vi "S2C_5190CR_Proc_SetOutput.vi"(7 "Local?":bool, 8 "Error In":errorcluster, 10 "Command":string, 11 "JSON String":string) -> (0 "Error Out":errorcluster, 3 "Response":variant)   [LabVIEW 2015]
doc: "Configures the state of an outlet."
uses:
  S2C_5190CR_Proc_Globals.vi
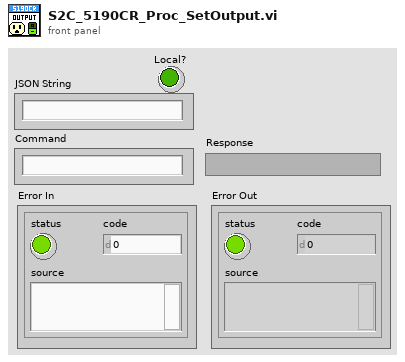
[diagram p1: front panel]
types:
  T1 = cluster{"OutletPlug":u16, "OutletState":bool, "PowerOnDelay(ms)":u32, "PowerOffDelay(ms)":u32, "WaitOnState":bool, "Timeout(ms)":i32}
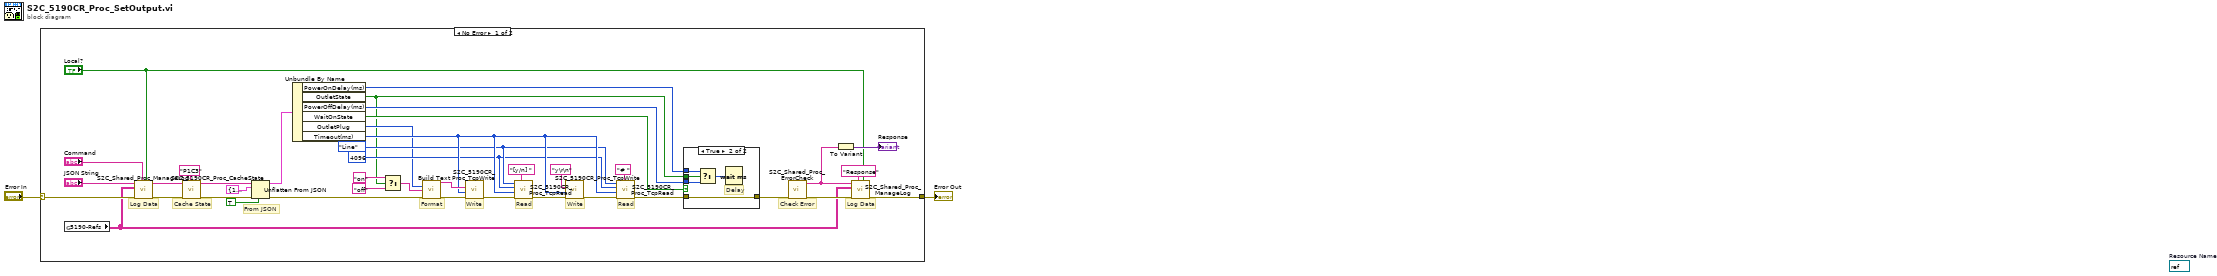
[diagram p0: block diagram]
diagram:
  (unwired) refnum<visa-resource-name> refnum  # Resource Name
  n1 = case shown="No Error" "Error In" {
    selector: "Error In" -> [w40 w49]
    tunnel: [w31 w49] -> w1
    frame No Error {
      w16 = enum16{"Normal", "Line"}."Line" ("Read Mode")
      w15 = 4096 ("Bytes")
      # "Read"
      # "Write"
      # "Read"
      # "Check Error"
      # "Write"
      # "Format"
      # "Cache State"
      # "Log Data"
      # "Log Data"
      # "From JSON"
      n2 = global read "S2C_5190CR_Proc_Globals.vi" "5190-Refs"() -> (w24:string[][])
      n3 = call "S2C_Shared_Proc_ManageLog.vi"("Local?"="Local?", "Command"="Command", "Error In"=w40, "Refs"=w24, "Data In"="JSON String") -> ("Error Out"=w36:errorcluster, "Data Out"=w35:string)  [unwired: 5 in]
      n4 = call "S2C_5190CR_Proc_CacheState.vi"("Label"="P1C3", "Error In"=w36, "Data In"=w35) -> ("Error Out"=w33:errorcluster, "Data Out"=w34:string)  [unwired: 7 in]
      n5 = Unflatten From JSON(JSON string=w34, type and defaults=T1 {"OutletPlug"=1, "OutletState"=TRUE, "PowerOnDelay(ms)"=50, "PowerOffDelay(ms)"=0, "WaitOnState"=TRUE, "Timeout(ms)"=10000} ("P1C3"), default null elements? (F)=TRUE, error in (no error)=w33) -> (value=w30:T1, error out=w29:errorcluster)  [unwired: 3 in]
      n6 = Unbundle By Name(w30) -> ("PowerOnDelay(ms)"=w12:u32, "OutletState"=w5:bool, "PowerOffDelay(ms)"=w6:u32, "WaitOnState"=w7:bool, "OutletPlug"=w8:u16, "Timeout(ms)"=w17:i32)
      n7 = Select(t="on" ("string"), s=w5, f="off" ("string")) -> (s? t:f=w9:string)
      n8 = call "Build Text"("Outlet"=w8, "State"=w9, "error in (no error)"=w29) -> ("Result"=w22:string, "error out"=w28:errorcluster)  [unwired: 11 in]
      n9 = call "S2C_5190CR_Proc_TcpWrite.vi"("Error In"=w28, "Timeout(ms)"=w17, "Data"=w22) -> ("Error Out"=w27:errorcluster)  [unwired: 8 in]
      n10 = call "S2C_5190CR_Proc_TcpRead.vi"("Line Seperator"="[y/n] " ("line separator"), "Error In"=w27, "Timeout(ms)"=w17, "Bytes"=w15, "Read Mode"=w16) -> ("Error Out"=w20:errorcluster)  [unwired: 5 in, 1 out]
      n11 = call "S2C_5190CR_Proc_TcpWrite.vi"("Error In"=w20, "Timeout(ms)"=w17, "Data"="y\r\n" ("data in")) -> ("Error Out"=w18:errorcluster)  [unwired: 8 in]
      n12 = call "S2C_5190CR_Proc_TcpRead.vi"("Line Seperator"="# " ("line separator"), "Error In"=w18, "Timeout(ms)"=w17, "Bytes"=w15, "Read Mode"=w16) -> ("Error Out"=w13:errorcluster)  [unwired: 5 in, 1 out]
      n13 = case shown="True" w7 {
        tunnel: w13 -> [w43 w45]
        tunnel: w6 -> [_ w47]
        tunnel: w12 -> [_ w48]
        tunnel: w5 -> [_ w46]
        tunnel: [w43 w45] -> w4
        frame False {
        }
        frame True {
          # "Delay"
          n14 = Select(t=w48, s=w46, f=w47) -> (s? t:f=w44:u32)
          n15 = Wait (ms)(milliseconds to wait=w44) -> ()  [unwired: 1 out]
        }
      }
      n16 = call "S2C_Shared_Proc_ErrorCheck.vi"("Error In"=w4) -> ("Error Out"=w26:errorcluster, "Status"=w25:string)  [unwired: 9 in]
      n17 = To Variant(anything=w25) -> (Variant=→"Response":variant)
      n18 = call "S2C_Shared_Proc_ManageLog.vi"("Local?"="Local?", "Command"="Response", "Error In"=w26, "Refs"=w24, "Data In"=w25) -> ("Error Out"=w31:errorcluster)  [unwired: 5 in, 1 out]
    }
    frame Error {
    }
  }
  "Error Out" <- w1
